vi "Get Cursor Position.vi"(2 "Cursor ID":u32, 3 "Graph Reference":refnum<vi>) -> (0 "X Position":dbl, 1 "Y Position":dbl)   [LabVIEW 2013]
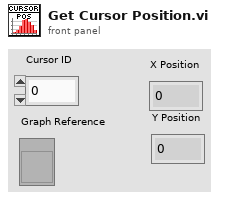
[diagram p1: front panel]
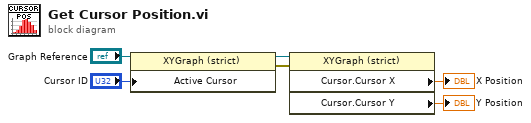
[diagram p0: block diagram]
diagram:
  n1 = property class="XYGraph (strict)"(reference="Graph Reference", "Active Cursor"="Cursor ID") -> (reference out=w3:refnum<vi>, error out=w2:errorcluster)  [unwired: 1 in]
  n2 = property class="XYGraph (strict)"(reference=w3, error in=w2) -> ("Cursor.Cursor X"=→"X Position":dbl, "Cursor.Cursor Y"=→"Y Position":dbl)  [unwired: 2 out]
